vi "Waveform Output.vi"(8 "error in (no error)":errorcluster, 11 "Node Ptr":T1 format="%.0x") -> (0 "error out":errorcluster)   [LabVIEW 2019, in "FPGA Addon System Explorer.lvlib"]
uses:
  FPGA Addon System Explorer.lvlib
  <vilib>/NI VeriStand/Custom Device API/Custom Device API.lvlib
  <vilib>/NI VeriStand/UI Controls/Single Node Browser/NI_VS UI Single Node Browser.lvlib
  NationalInstruments.VeriStand.SystemStorageUI
  <vilib>/NI VeriStand/Custom Device API/Get Item Property (Dependent Node Pointer).vi
  NationalInstruments.VeriStand.SystemStorage
  Addon Shared/Constants.vi
  Addon Shared/FPGA Addon Shared.lvlib
  <vilib>/NI VeriStand/Custom Device API/Set Item Property (Dependent Node Pointer).vi
  <vilib>/NI VeriStand/Custom Device API/Custom Device Item Ref.ctl
panel:
  out "Original Name":string
  in  "Source Waveform":refnum<k24>(container)
  in  "Header":cluster{"Section Name":string}={"Section Name"="Custom Device Item Settings"}
  in  "Description":string
  in  "Name":string
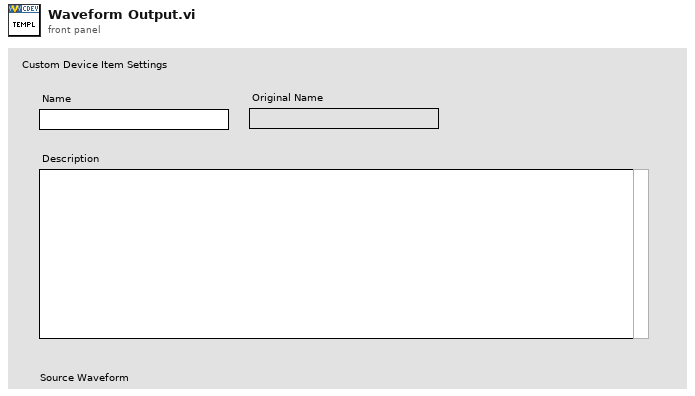
[diagram p1: front panel]
types:
  T1 = typedef "Custom Device API.lvlib/Custom Device Item Ref.ctl" = u64
  T2 = typedef "Custom Device API.lvlib/Custom Device Pointer.ctl" = refnum<k24>
  T3 = typedef "Custom Device API.lvlib/Custom Device Item Info.ctl" = cluster{"Name":string, "Is Channel":bool, "GUID":string, "Is Waveform":bool}
  T4 = typedef "NI_VS UI Single Node Browser.lvlib/Callback Type.ctl" = cluster{"Net Callbacks":refnum<k27>[], "Event":refnum<user-event>}
  T5 = typedef "Custom Device API.lvlib/Custom Device Commands.ctl" = enum16{"Default", "Item renamed", "Shutdown", "Dynamic button pressed"}
  T6 = typedef "NI_VS UI Single Node Browser.lvlib/Node Ref.ctl" = refnum<k24>
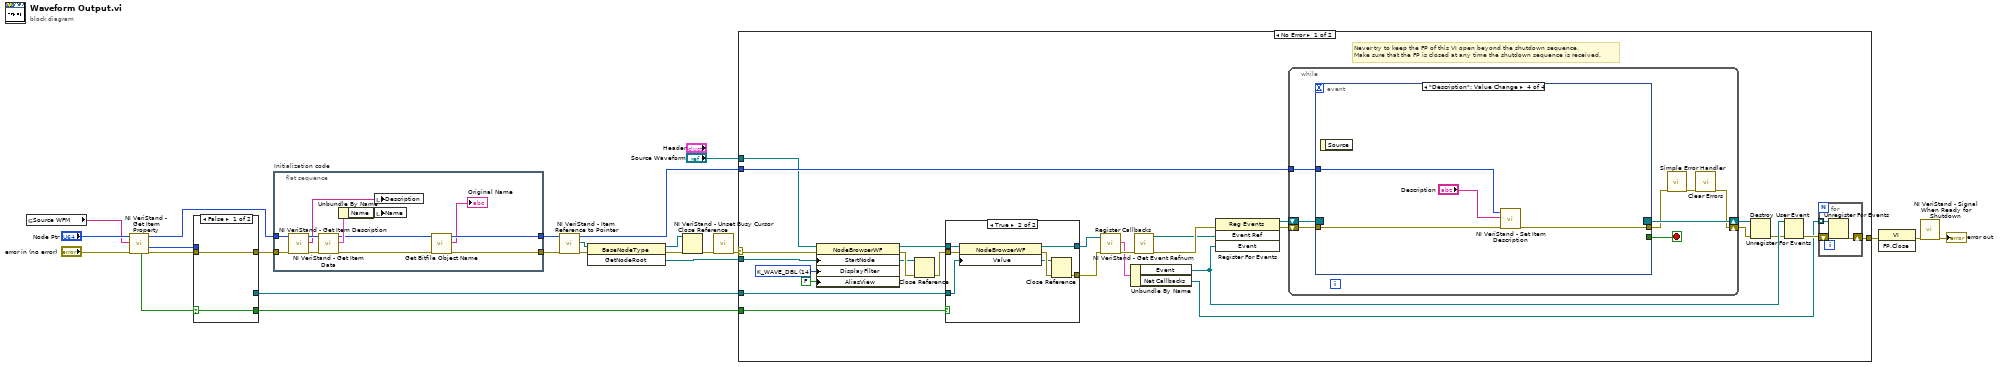
[diagram p0: block diagram]
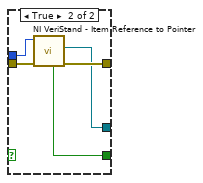
[diagram p2: hidden frame]
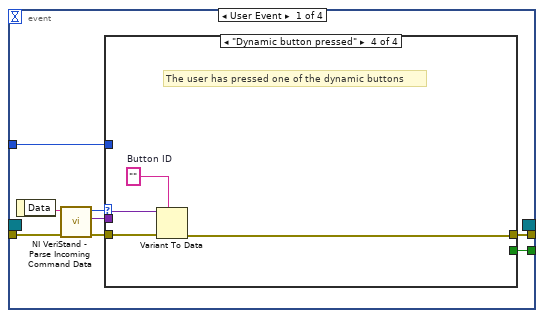
[diagram p4: hidden frame]
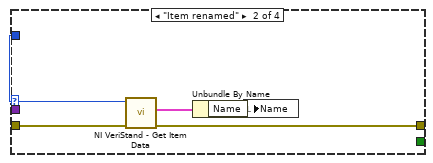
[diagram p6: hidden frame]
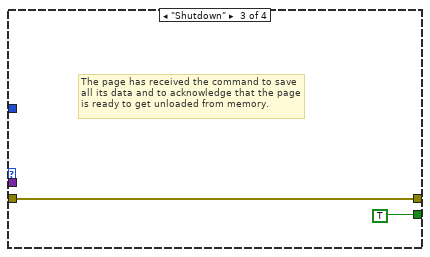
[diagram p7: hidden frame]
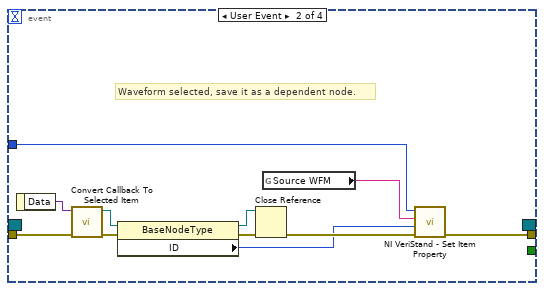
[diagram p8: hidden frame]
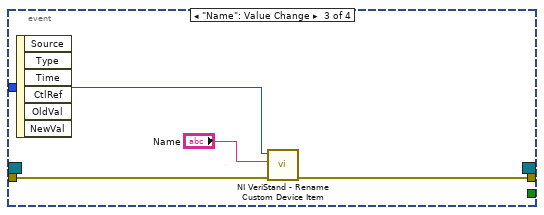
[diagram p9: hidden frame]
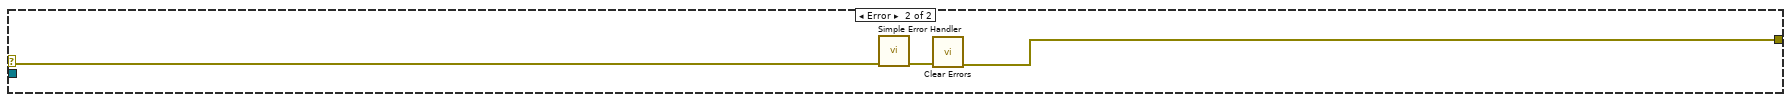
[diagram p10: hidden frame]
diagram:
  n1 = global read "Constants.vi" "Source WFM"() -> (w1:string)
  n2 = call-poly <vilib>:"NI VeriStand - Get Item Property.vi"("error in (no error)"="error in (no error)", "Property Name"=w1, "Item Ref in"="Node Ptr") -> ("error out"=w13:errorcluster, "Dependent Node Ref"=w12:T1, "Item Ref out"=w5:T1, "Found"=w11:bool)  [unwired: 5 in]
  n3 = case shown="False" w11 {
    selector: w11 -> [w25 _]
    tunnel: [w26 w31] -> w6
    tunnel: [_ w30] -> w14
    tunnel: w13 -> [w26 w29]
    tunnel: w12 -> [_ w28]
    tunnel: [w25 w27] -> w10
    frame False {
    }
    frame True {
      n4 = call <vilib>:"NI VeriStand - Item Reference to Pointer.vi"("error in (no error)"=w29, "Item Ref in"=w28) -> ("error out"=w31:errorcluster, "Node Pointer"=w30:T2, "Found"=w27:bool)  [unwired: 6 in, 1 out]
    }
  }
  n5 = flat-sequence "Initialization code" {
    tunnel: w6 -> [w42]
    tunnel: w5 -> [w41]
    tunnel: [w35] -> w4
    tunnel: [w33] -> w3
    frame #0 {
      n6 = call <vilib>:"NI VeriStand - Get Item Description.vi"("error in (no error)"=w42, "Item Ref in"=w41) -> ("error out"=w39:errorcluster, "Description"=w40:string, "Item Ref out"=w43:T1)  [unwired: 7 out]
      n7 = call <vilib>:"NI VeriStand - Get Item Data.vi"("error in (no error)"=w39, "Item Ref in"=w43) -> ("error out"=w36:errorcluster, "Item Info"=w38:T3, "Item Ref out"=w34:T1)  [unwired: 7 out]
      n8 = Unbundle By Name(w38) -> ("Name"=w37:string)
      n9 = local write "Description"(w40) -> ()
      n10 = local write "Name"(w37) -> ()
      n11 = call "Get Bitfile Object Name.vi"("error in (no error)"=w36, "Item Ref in"=w34) -> ("error out"=w35:errorcluster, "Value"=→"Original Name":string, "Item Ref out"=w33:T1)  [unwired: 7 in]
    }
  }
  n12 = call <vilib>:"NI VeriStand - Item Reference to Pointer.vi"("error in (no error)"=w4, "Item Ref in"=w3) -> ("error out"=w19:errorcluster, "Node Pointer"=w20:T2, "Item Ref out"=w21:T1)  [unwired: 6 in, 1 out]
  n13 = invoke class="BaseNodeType" method="GetNodeRoot"(reference=w20, error in=w19) -> (reference out=w15:T2, error out=w16:errorcluster, "GetNodeRoot"=w18:refnum<k24>)  [unwired: 1 in]
  n14 = Close Reference(reference=w15, error in (no error)=w16) -> (error out=w17:errorcluster)
  n15 = call <vilib>:"NI VeriStand - Unset Busy Cursor.vi"("error in (no error)"=w17) -> ("error out"=w22:errorcluster)  [unwired: 10 out]
  n16 = case shown="No Error" w22 {
    selector: w22 -> [w58 w130]
    tunnel: [w52 w128] -> w24
    tunnel: w21 -> [w63 _]
    tunnel: w18 -> [w56 _]
    tunnel: w14 -> [w46 _]
    tunnel: w10 -> [w45 _]
    tunnel: "Source Waveform" -> [w44 _]
    frame No Error {
      w60 = u8 14 items=["K_CHAN_R", "K_CHAN_W", "K_CHAN_RW", "K_CHAN_VOLT", "K_CHAN_FAULT", "K_ALL", "K_CUSTOM", "K_CHAN_R_VIS", "K_CHAN_W_VIS", "K_CHAN_RW_VIS", "K_CHAN_VOLT_VIS", "K_CHAN_FAULT_VIS", "K_WAVE", "K_WAVE_VIS", "K_WAVE_DBL", "K_WAVE_CDB", "K_WAVE_DBL_VIS", "K_WAVE_CDB_VIS"] ("DisplayFilter")
      # "Never try to keep the FP of this VI open beyond the shutdown sequence.\nMake sure that the FP is closed at any time the shutdown sequence is received."
      n17 = property class="NodeBrowserWF"(reference=w44, error in=w58, "StartNode"=w56, "DisplayFilter"=w60, "AliasView"=FALSE) -> (reference out=w48:refnum<k24>, error out=w57:errorcluster)
      n18 = Close Reference(reference=w56, error in (no error)=w57) -> (error out=w49:errorcluster)
      n19 = case shown="True" w45 {
        tunnel: [w70 w77] -> w50
        tunnel: w49 -> [w70 w76]
        tunnel: w48 -> [w71 w75]
        tunnel: [w71 w73] -> w47
        tunnel: w46 -> [_ w72]
        frame False {
        }
        frame True {
          n20 = property class="NodeBrowserWF"(reference=w75, error in=w76, "Value"=w72) -> (reference out=w73:refnum<k24>, error out=w74:errorcluster)
          n21 = Close Reference(reference=w72, error in (no error)=w74) -> (error out=w77:errorcluster)
        }
      }
      n22 = call <vilib>:"Register Callbacks.vi"("error in (no error)"=w50, "Single Node Browser"=w47) -> ("error out"=w62:errorcluster, "Callbacks"=w61:T4)  [unwired: 7 in, 1 out]
      n23 = Unbundle By Name(w61) -> ("Event"=w55:refnum<user-event>, "Net Callbacks"=w51:refnum<k27>[])
      n24 = call <vilib>:"NI VeriStand - Get Event Refnum.vi"("error in (no error)"=w62) -> ("error out"=w69:errorcluster, "Event Ref"=w66:refnum<user-event>)  [unwired: 9 out]
      n25 = register-events(error in=w69, w66, w55) -> (reference out=w64:refnum<event-registration>, error out=w65:errorcluster)  [unwired: 1 in]
      n26 = while {
        tunnel: w63 -> [w84]
        shift-right: [w81] -> w67
        shift-left: w65 -> [w87]
        shift-right: [w88] -> w68
        shift-left: w64 -> [w86]
        stop <- w85 stop-if-true
        n27 = event shown="[3] \"Description\": Value Change" {
          selector: w86 -> [_ _ _ _]
          dyn-events: [_ _ _ _] -> w88
          timeout: _ -> [_ _ _ _]
          tunnel: w87 -> [w96 w119 w123 w126]
          tunnel: [w92 _ _ _] -> w85
          tunnel: [w91 w112 w122 w125] -> w83
          tunnel: w84 -> [w90 w113 w121 w127]
          event User Event {
            n28 = event-data() -> ("Data"=w95:string)  [unwired: 1 out]
            n29 = call <vilib>:"NI VeriStand - Parse Incoming Command Data.vi"("error in (no error)"=w96, "Incoming data"=w95) -> ("error out"=w94:errorcluster, "Outgoing data"=w89:variant, "Action"=w93:T5)  [unwired: 7 out]
            n30 = case shown="\"Dynamic button pressed\"" w93 {
              tunnel: w94 -> [w97 w102 w103 w108]
              tunnel: [_ _ TRUE _] -> w92
              tunnel: [w97 w99 w103 w105] -> w91
              tunnel: w90 -> [_ w101 _ _]
              tunnel: w89 -> [_ _ _ w107]
              frame "Default", Default {
              }
              frame "Item renamed" {
                n31 = call <vilib>:"NI VeriStand - Get Item Data.vi"("error in (no error)"=w102, "Item Ref in"=w101) -> ("error out"=w99:errorcluster, "Item Info"=w100:T3)  [unwired: 8 out]
                n32 = Unbundle By Name(w100) -> ("Name"=w98:string)
                n33 = local write "Name"(w98) -> ()
              }
              frame "Shutdown" {
                # "The page has received the command to save all its data and to acknowledge that the page is ready to get unloaded from memory."
              }
              frame "Dynamic button pressed" {
                w106 = ""  # Button ID
                # "The user has pressed one of the dynamic buttons"
                n34 = Variant To Data(error in=w108, type=w106, Variant=w107) -> (error out=w105:errorcluster)  [unwired: 1 out]
              }
            }
          }
          event User Event {
            # "Waveform selected, save it as a dependent node."
            n35 = event-data() -> ("Data"=w118:variant)  [unwired: 1 out]
            n36 = call <vilib>:"Convert Callback To Selected Item.vi"("error in"=w119, "Data"=w118) -> ("error out"=w117:errorcluster, "Selected Item"=w116:T6)  [unwired: 8 in]
            n37 = property class="BaseNodeType"(reference=w116, error in=w117) -> (reference out=w114:T6, error out=w115:errorcluster, "ID"=w110:u64)
            n38 = Close Reference(reference=w114, error in (no error)=w115) -> (error out=w111:errorcluster)
            n39 = global read "Constants.vi" "Source WFM"() -> (w109:string)
            n40 = call-poly <vilib>:"NI VeriStand - Set Item Property.vi"("error in (no error)"=w111, "Dependent Node Ref"=w110, "Property Name"=w109, "Item Ref in"=w113) -> ("error out"=w112:errorcluster)  [unwired: 5 in, 2 out]
          }
          event "Name": Value Change {
            n41 = event-data() -> ()  [unwired: 7 out]
            n42 = call <vilib>:"NI VeriStand - Rename Custom Device Item.vi"("error in (no error)"=w123, "New Name"="Name", "Item Ref in"=w121) -> ("error out"=w122:errorcluster)  [unwired: 1 in, 7 out]
          }
          event "Description": Value Change {
            n43 = event-data() -> ()  [unwired: 2 out]
            n44 = call <vilib>:"NI VeriStand - Set Item Description.vi"("error in (no error)"=w126, "Description"="Description", "Item Ref in"=w127) -> ("error out"=w125:errorcluster)  [unwired: 8 out]
          }
        }
        n45 = call <vilib>:"Simple Error Handler.vi"("error in (no error)"=w83) -> ("error out"=w82:errorcluster)  [unwired: 1 in, 7 out]
        n46 = call <vilib>:"Clear Errors.vi"("error in (no error)"=w82) -> ("error out"=w81:errorcluster)  [unwired: 1 in, 5 out]
      }
      n47 = Unregister For Events(event registration refnum=w68, error in=w67) -> (error out=w54:errorcluster)
      n48 = Destroy User Event(user event=w55, error in=w54) -> (error out=w53:errorcluster)
      n49 = for {
        tunnel: w51 -> [w78] mode=indexing
        shift-right: [w79] -> w52
        shift-left: w53 -> [w80]
        n50 = Unregister For Events(event registration refnum=w78, error in=w80) -> (error out=w79:errorcluster)
      }
    }
    frame Error {
      n51 = call <vilib>:"Simple Error Handler.vi"("error in (no error)"=w130) -> ("error out"=w129:errorcluster)  [unwired: 1 in, 7 out]
      n52 = call <vilib>:"Clear Errors.vi"("error in (no error)"=w129) -> ("error out"=w128:errorcluster)  [unwired: 1 in, 5 out]
    }
  }
  n53 = invoke class="VI" method="FP.Close"(error in=w24) -> (error out=w23:errorcluster)  [unwired: 2 in, 2 out]
  n54 = call <vilib>:"NI VeriStand - Signal When Ready for Shutdown.vi"("error in (no error)"=w23) -> ("error out"=→"error out":errorcluster)  [unwired: 10 out]
